vi "LanchAngleAndSpeed_with DRAG.vi"(2 "basket number":i32, 3 "distance to center of basket (x axies)":dbl) -> (0 "speed":dbl, 1 "angle":dbl)   [LabVIEW 2011]
panel:
  # "3-top\n2-middle\n1-bottom"
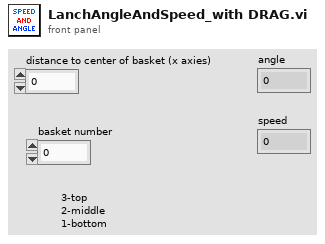
[diagram p1: front panel]
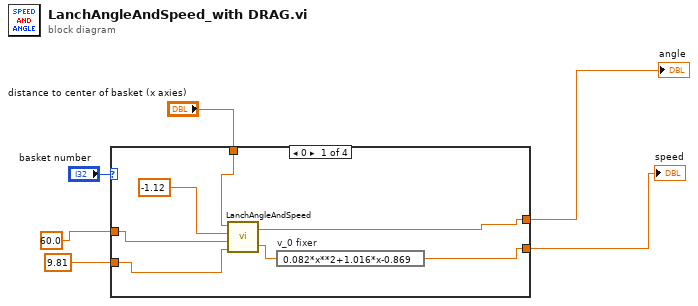
[diagram p0: block diagram]
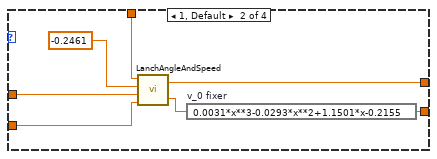
[diagram p2: hidden frame]
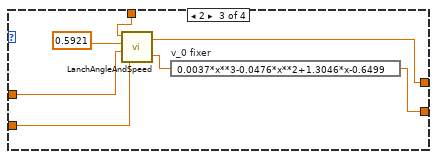
[diagram p3: hidden frame]
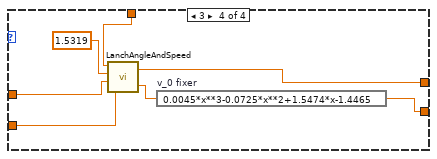
[diagram p4: hidden frame]
diagram:
  n1 = case shown="0" "basket number" {
    tunnel: "distance to center of basket (x axies)" -> [w11 w19 w26 w33]
    tunnel: 60.0 ("b") -> [w10 w18 w24 w31]
    tunnel: 9.81 ("g") -> [w9 w17 w23 w30]
    tunnel: [w8 w16 w22 w29] -> w2
    tunnel: [w7 w14 w21 w28] -> w1
    frame 0 {
      n2 = call "LanchAngleAndSpeed.vi"("g"=w9, "entry angle"=w10, "height"=-1.12, "horizontal distance"=w11) -> ("speed"=w12:dbl, "angle"=w8:dbl)
      n3 = expression code="0.082*x**2+1.016*x-0.869" "v_0 fixer"(w12) -> (w7:dbl)
    }
    frame 1, Default {
      n4 = call "LanchAngleAndSpeed.vi"("g"=w17, "entry angle"=w18, "height"=-0.2461, "horizontal distance"=w19) -> ("speed"=w15:dbl, "angle"=w16:dbl)
      n5 = expression code="0.0031*x**3-0.0293*x**2+1.1501*x-0.2155" "v_0 fixer"(w15) -> (w14:dbl)
    }
    frame 2 {
      n6 = call "LanchAngleAndSpeed.vi"("g"=w23, "entry angle"=w24, "height"=0.5921, "horizontal distance"=w26) -> ("speed"=w27:dbl, "angle"=w22:dbl)
      n7 = expression code="0.0037*x**3-0.0476*x**2+1.3046*x-0.6499" "v_0 fixer"(w27) -> (w21:dbl)
    }
    frame 3 {
      n8 = call "LanchAngleAndSpeed.vi"("g"=w30, "entry angle"=w31, "height"=1.5319, "horizontal distance"=w33) -> ("speed"=w34:dbl, "angle"=w29:dbl)
      n9 = expression code="0.0045*x**3-0.0725*x**2+1.5474*x-1.4465" "v_0 fixer"(w34) -> (w28:dbl)
    }
  }
  "angle" <- w2
  "speed" <- w1
